vi "Read Log File Path.vi"(8 "error in (no error)":errorcluster, 11 "Abstract Log Consumer in":refnum<class "Abstract Log Consumer.lvclass">) -> (0 "error out":errorcluster, 2 "Log File Path":path, 3 "Abstract Log Consumer out":refnum<class "Abstract Log Consumer.lvclass">)   [LabVIEW 2020]
uses:
  Abstract Log Consumer.lvclass
  Abstract Log Consumer.lvclass/Abstract Log Consumer.ctl
  C:/git/buckd/niveristand-custom-device-message-library/Source/Consumer/Abstract Consumer/Abstract Consumer.lvclass
  C:/git/buckd/niveristand-custom-device-message-library/Source/Log/Abstract Log Consumer/Abstract Log Consumer.lvclass
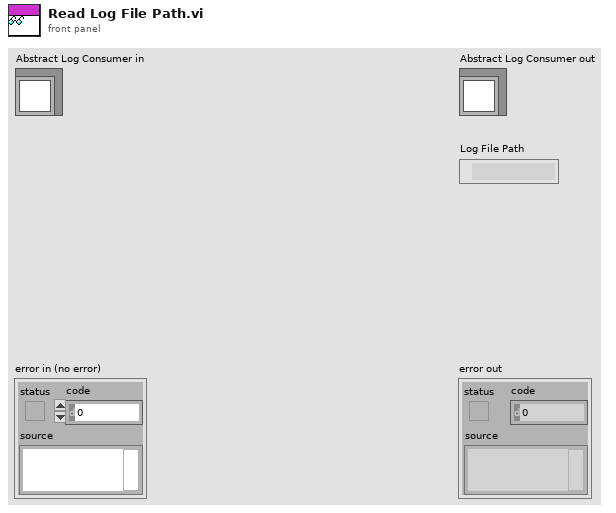
[diagram p1: front panel]
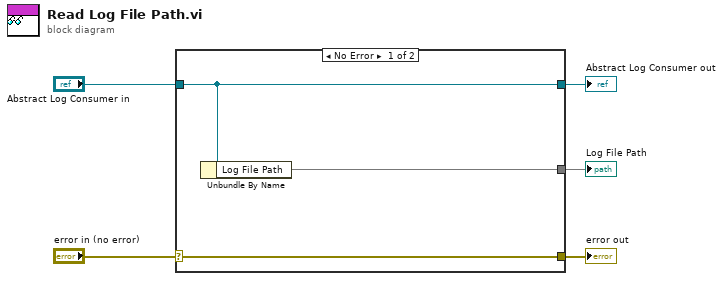
[diagram p0: block diagram]
diagram:
  n1 = case shown="No Error" "error in (no error)" {
    selector: "error in (no error)" -> [w8 w9]
    tunnel: [w8 w9] -> w4
    tunnel: [w7 w10] -> w2
    tunnel: "Abstract Log Consumer in" -> [w7 w10]
    tunnel: [w6 _] -> w1
    frame No Error {
      n2 = Unbundle By Name(w7) -> ("Log File Path"=w6)
    }
    frame Error {
    }
  }
  "error out" <- w4
  "Abstract Log Consumer out" <- w2
  "Log File Path" <- w1
